vi "CSMSVMgr Mark All Temp Variables as Permanent.vi"(8 "error in (no error)":errorcluster, 10 "Path":path, 11 "CSM-Static-Variable-Manager in":refnum<class "CSM-Static-Variable-Manager.lvclass">) -> (0 "error out":errorcluster, 3 "CSM-Static-Variable-Manager out":refnum<class "CSM-Static-Variable-Manager.lvclass">)   [LabVIEW 2017, in "INI-Static-Variable-Support.lvlib" / "CSM-Static-Variable-Manager.lvclass"]
uses:
  CSM-Static-Variable-Manager.lvclass
  CSM-Static-Variable-Manager.lvclass/CSM-Static-Variable-Manager.ctl
  LabVIEW-Config/Config.ctl
  LabVIEW-Config/LineToken.ctl
  LabVIEW-Config/LabVIEW-Config.lvlib
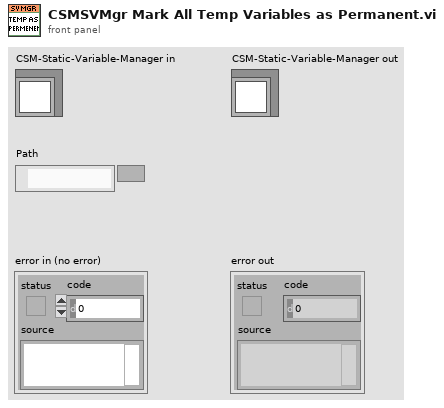
[diagram p1: front panel]
types:
  T1 = typedef "LabVIEW-Config.lvlib/Config.ctl" = cluster{"Path":path, "Lines":string[], "Tokens":T2[], "Modified?":bool}
  T2 = typedef "LabVIEW-Config.lvlib/LineToken.ctl" = enum8{"comment", "section", "key", "more"}
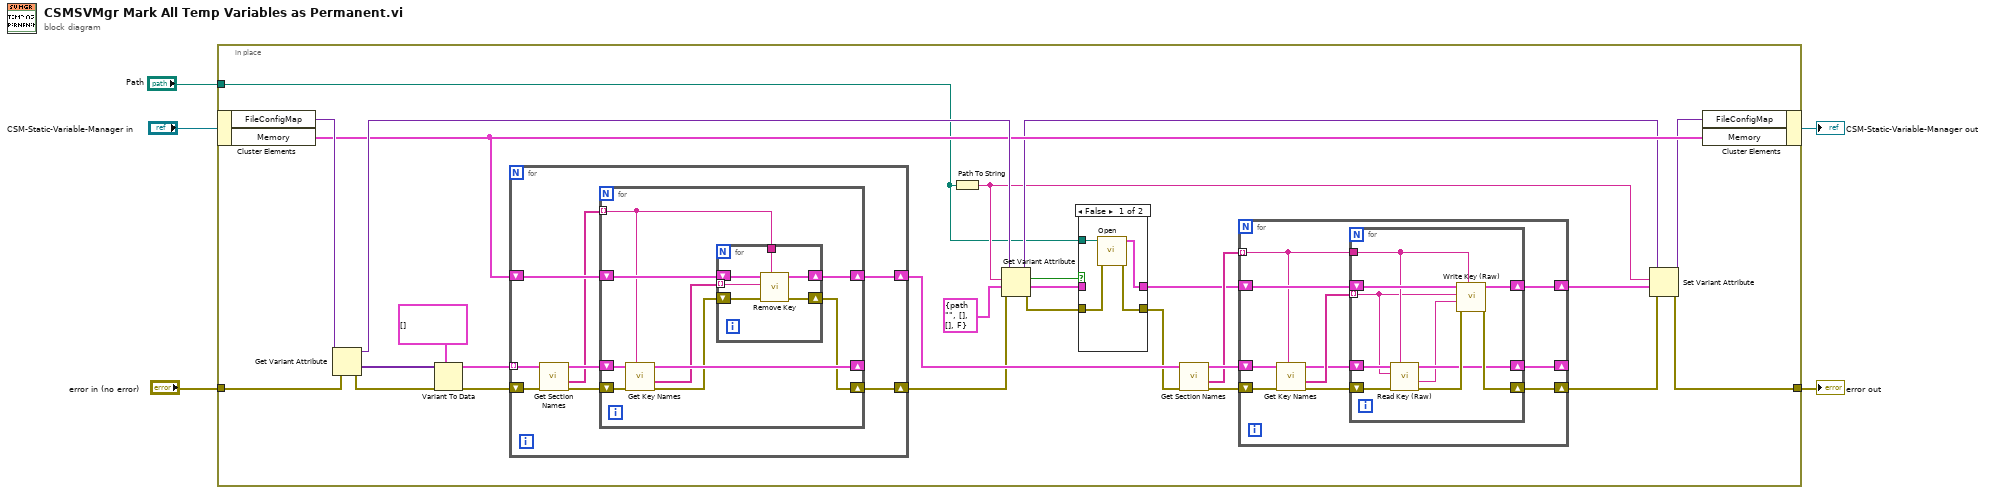
[diagram p0: block diagram]
diagram:
  n1 = in-place {
    in-place-border: "error in (no error)" -> [w29]
    in-place-border: [w12] -> w2
    in-place-border: "Path" -> [w11]
    n2 = in-place-cluster #1("CSM-Static-Variable-Manager in") -> ("FileConfigMap"=w32:variant, "Memory"=w24:T1)
    n3 = Get Variant Attribute(Variant=w32, error in=w29) -> (duplicate Variant=w25:variant, values=w31:variant[], error out=w30:errorcluster)  [unwired: 2 in, 1 out]
    n4 = Variant To Data(error in=w30, type=T1[] [], Variant=w31) -> (data=w26:T1[], error out=w28:errorcluster)
    n5 = for {
      shift-right: [w64] -> w23
      shift-left: w24 -> [w65]
      shift-right: [w59] -> w18
      shift-left: w28 -> [w62]
      tunnel: w26 -> [w66] mode=indexing
      n6 = call "Get Section Names.vi"("error in (no error)"=w62, "Config in"=w66) -> ("error out"=w61:errorcluster, "Section Names"=w60:string[], "Config out"=w63:T1)  [unwired: 7 in]
      n7 = for {
        shift-right: [w71] -> w64
        shift-left: w65 -> [w72]
        shift-right: [w68] -> w59
        shift-left: w61 -> [w73]
        tunnel: w60 -> [w70] mode=indexing
        shift-right: [w75] -> _
        shift-left: w63 -> [w74]
        n8 = call "Get Key Names.vi"("Section Name"=w70, "error in (no error)"=w73, "Config in"=w74) -> ("error out"=w69:errorcluster, "Key Names"=w67:string[], "Config out"=w75:T1)  [unwired: 5 in, 1 out]
        n9 = for {
          tunnel: w70 -> [w79]
          tunnel: w67 -> [w76] mode=indexing
          shift-right: [w80] -> w71
          shift-left: w72 -> [w81]
          shift-right: [w77] -> w68
          shift-left: w69 -> [w78]
          n10 = call "Remove Key.vi"("Section Name"=w79, "error in (no error)"=w78, "Key Name"=w76, "Config in"=w81) -> ("error out"=w77:errorcluster, "Config out"=w80:T1)  [unwired: 5 in, 1 out]
        }
      }
    }
    n11 = Path To String(path=w11) -> (string=w15:string)
    n12 = Get Variant Attribute(Variant=w25, name=w15, default value (empty Variant)=T1 {"Path"=path "", "Lines"=[], "Tokens"=[], "Modified?"=FALSE} ("Config out"), error in=w18) -> (duplicate Variant=w19:variant, found=w7:bool, value=w6:T1, error out=w8:errorcluster)
    n13 = case shown="False" w7 {
      tunnel: w11 -> [w36 _]
      tunnel: [w35 w37] -> w10
      tunnel: [w34 w38] -> w9
      tunnel: w8 -> [w33 w38]
      tunnel: w6 -> [_ w37]
      frame False {
        n14 = call "Open.vi"("error in (no error)"=w33, "Path"=w36) -> ("error out"=w34:errorcluster, "Config"=w35:T1)  [unwired: 6 in, 2 out]
      }
      frame True {
      }
    }
    n15 = call "Get Section Names.vi"("error in (no error)"=w9, "Config in"=w23) -> ("error out"=w21:errorcluster, "Section Names"=w20:string[], "Config out"=w22:T1)  [unwired: 7 in]
    n16 = for {
      shift-right: [w42] -> w13
      shift-left: w21 -> [w47]
      tunnel: w20 -> [w45] mode=indexing
      shift-right: [w41] -> _
      shift-left: w22 -> [w48]
      shift-right: [w39] -> w14
      shift-left: w10 -> [w46]
      n17 = call "Get Key Names.vi"("Section Name"=w45, "error in (no error)"=w47, "Config in"=w48) -> ("error out"=w43:errorcluster, "Key Names"=w44:string[], "Config out"=w40:T1)  [unwired: 5 in, 1 out]
      n18 = for {
        tunnel: w45 -> [w52]
        tunnel: w44 -> [w51] mode=indexing
        shift-right: [w57] -> w42
        shift-left: w43 -> [w56]
        shift-right: [w54] -> w41
        shift-left: w40 -> [w53]
        shift-right: [w49] -> w39
        shift-left: w46 -> [w58]
        n19 = call "Read Key (Raw).vi"("Section Name"=w52, "error in (no error)"=w56, "Key Name"=w51, "Config in"=w53) -> ("error out"=w55:errorcluster, "Content"=w50:string, "Config out"=w54:T1)  [unwired: 4 in, 1 out]
        n20 = call "Write Key (Raw).vi"("Section Name"=w52, "error in (no error)"=w55, "Content"=w50, "Key Name"=w51, "Config in"=w58) -> ("error out"=w57:errorcluster, "Config out"=w49:T1)  [unwired: 4 in, 1 out]
      }
    }
    n21 = Set Variant Attribute(Variant=w19, name=w15, value=w14, error in=w13) -> (Variant out=w16:variant, error out=w12:errorcluster)  [unwired: 1 out]
    n22 = in-place-cluster #1("FileConfigMap"=w16, "Memory"=w24) -> (→"CSM-Static-Variable-Manager out":refnum<class "CSM-Static-Variable-Manager.lvclass">)
  }
  "error out" <- w2
